vi "UI Controller.vi"(8 "Error In":errorcluster) -> (0 "Error Out":errorcluster)   [LabVIEW 2019, in "Controller.lvlib"]
uses:
  Controller.lvlib
  User Event/Controls/UE Abort Action.ctl
  <vilib>/Utility/miscctls.llb/LVPointTypeDef.ctl
  Queues/Queues.lvlib
  Initialize/Initialize.lvlib
  UI/UI Main Page.vi
  UI/UIs.lvlib
panel:
  out "String":string
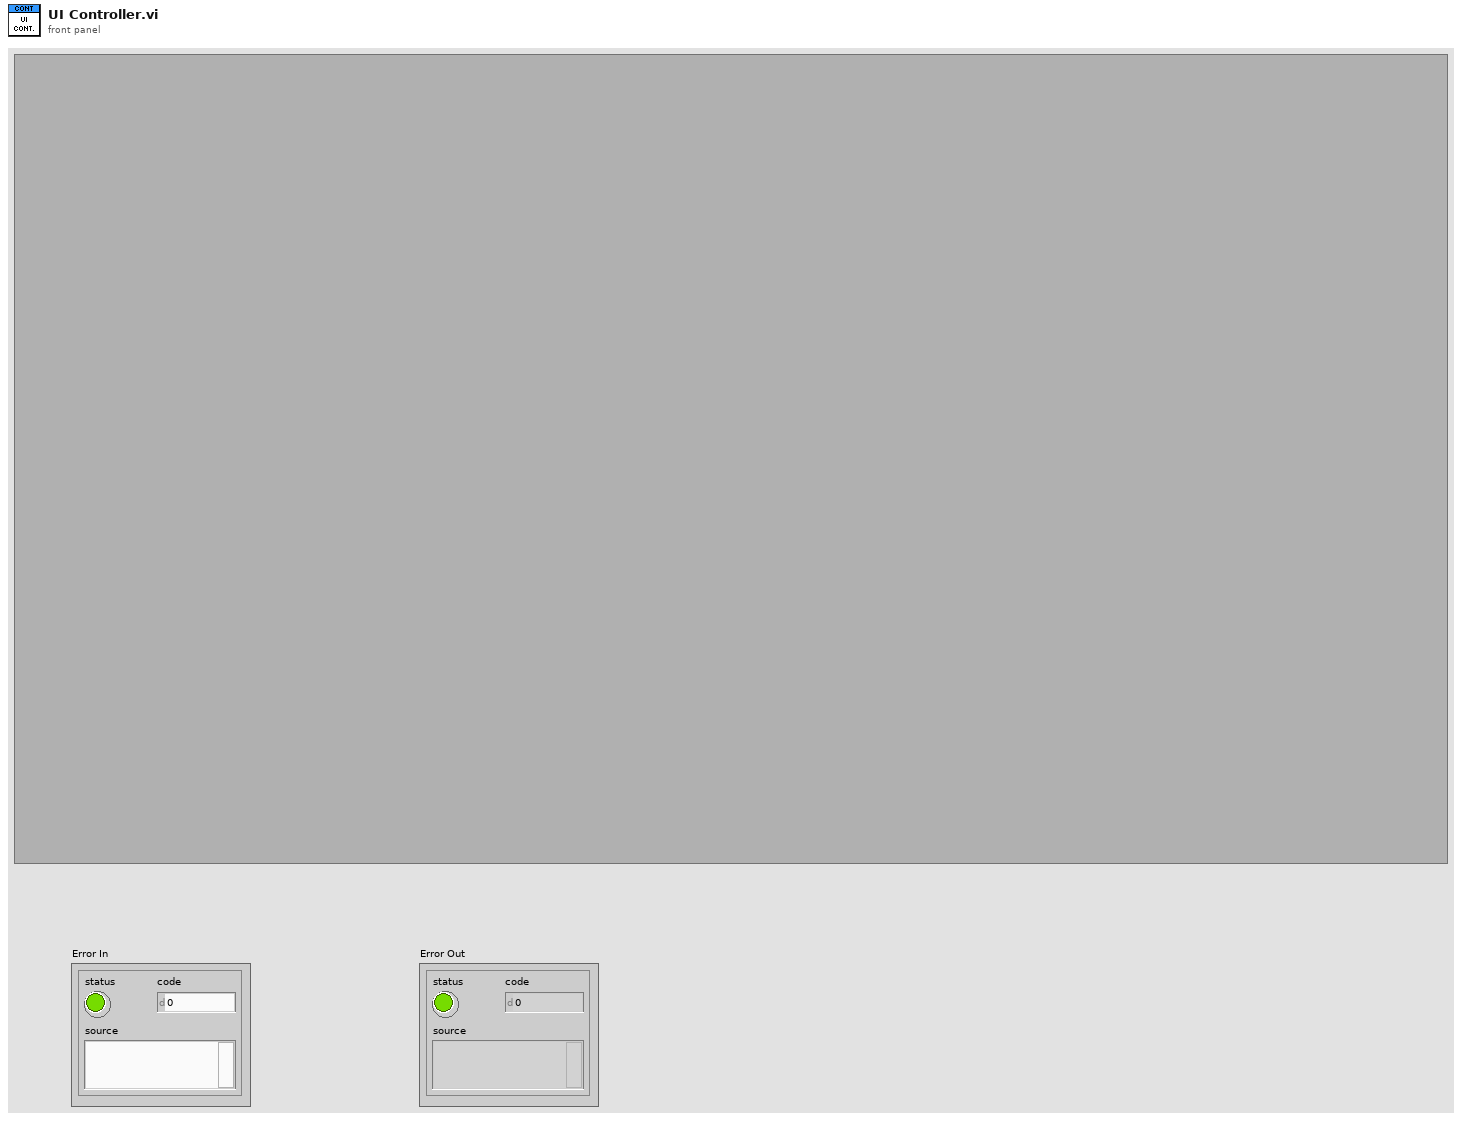
[diagram p1: front panel]
types:
  T1 = typedef "UE Abort Action.ctl" = enum16{"Create", "Get", "Destroy"}
  T2 = typedef "LVPointTypeDef.ctl" = cluster{"Horizontal":i16, "Vertical":i16}
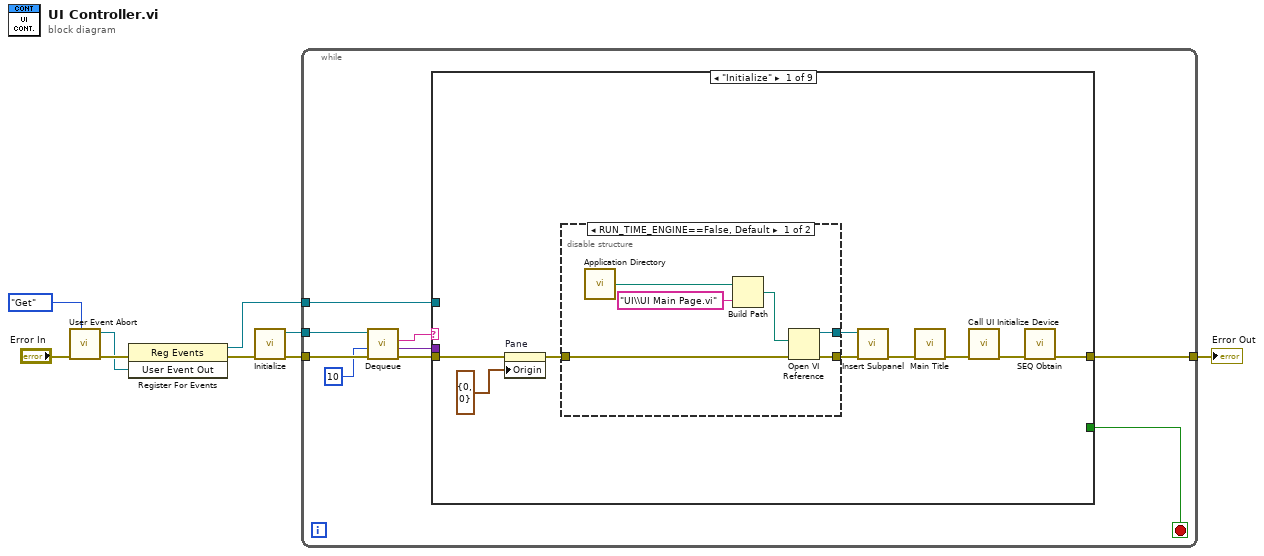
[diagram p0: block diagram]
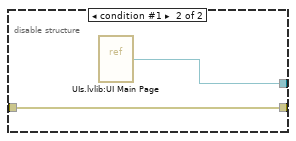
[diagram p2: hidden frame]
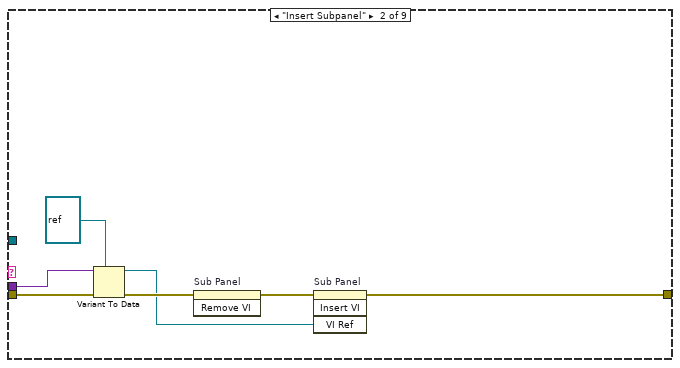
[diagram p3: hidden frame]
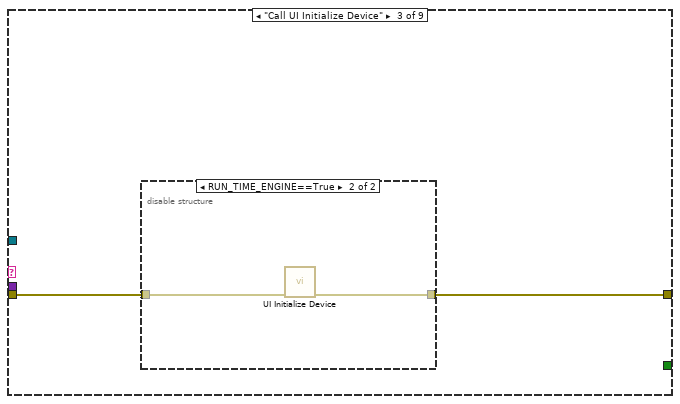
[diagram p4: hidden frame]
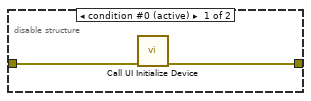
[diagram p5: hidden frame]
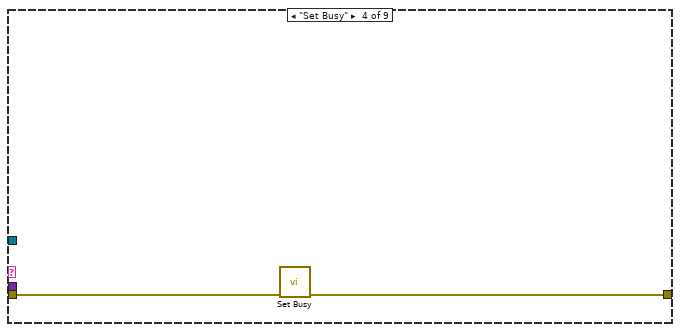
[diagram p6: hidden frame]
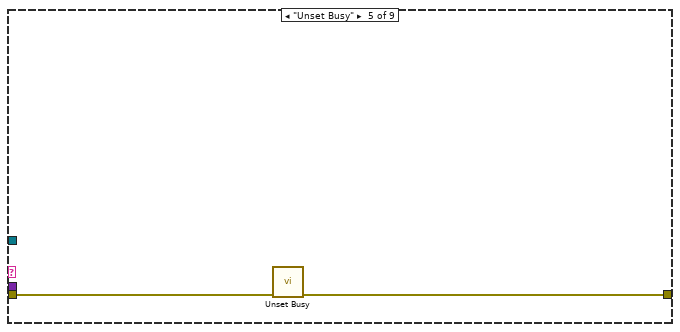
[diagram p7: hidden frame]
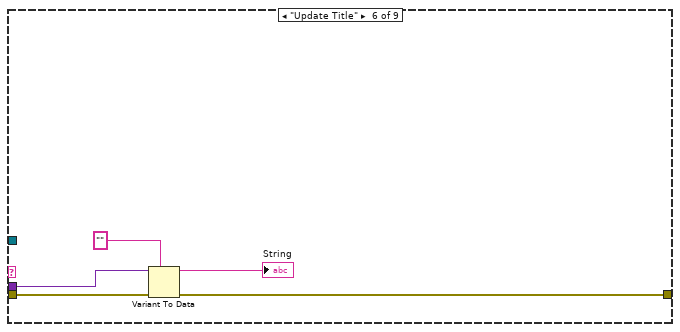
[diagram p8: hidden frame]
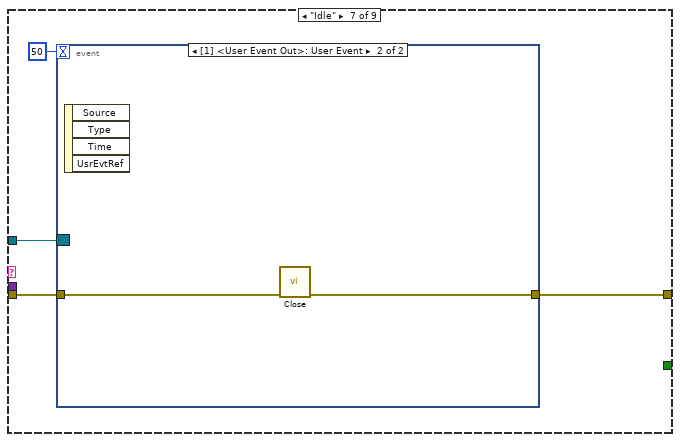
[diagram p9: hidden frame]
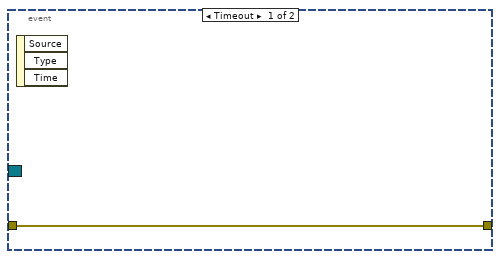
[diagram p10: hidden frame]
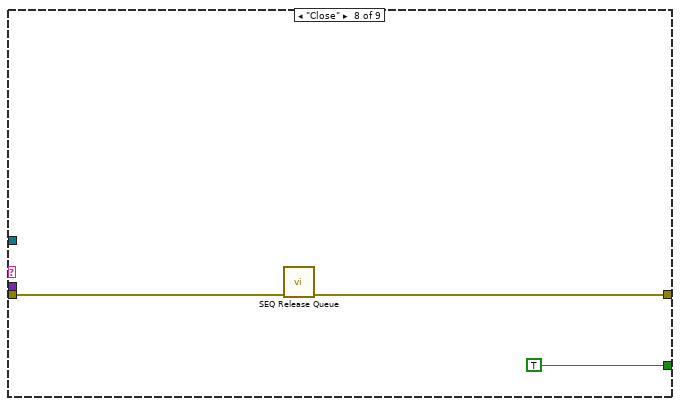
[diagram p11: hidden frame]
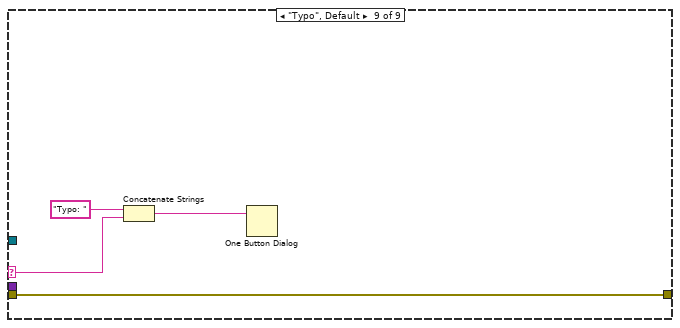
[diagram p12: hidden frame]
diagram:
  n1 = call "User Event Abort.vi"("Action"=UE_Abort_Action."Get", "Error In"="Error In") -> ("Error Out"=w4:errorcluster, "User Event Out"=w3:refnum<user-event>)  [unwired: 8 in]
  n2 = register-events(error in=w4, w3) -> (reference out=w1:refnum<event-registration>, error out=w2:errorcluster)  [unwired: 1 in]
  n3 = call "Initialize.vi"("Error In"=w2) -> ("Error Out"=w8:errorcluster, "Queue out"=w7:refnum<queue>)  [unwired: 9 in]
  n4 = while {
    tunnel: w7 -> [w18]
    tunnel: w8 -> [w17]
    tunnel: [w12] -> w9
    tunnel: w1 -> [w11]
    stop <- w10 stop-if-true
    n5 = call "Dequeue.vi"("Error In"=w17, "timeout in ms (-1)"=10, "Queue in"=w18) -> ("Error Out"=w16:errorcluster, "Data"=w14:variant, "State"=w15:string)  [unwired: 5 in, 1 out]
    n6 = case shown="\"Initialize\"" w15 {
      selector: w15 -> [_ _ _ _ _ _ _ _ w70]
      tunnel: w16 -> [w26 w42 w44 w50 w52 w57 w61 w66 w71]
      tunnel: [w21 w39 w43 w49 w51 w55 w59 w65 w71] -> w12
      tunnel: w14 -> [_ w38 _ _ _ w56 _ _ _]
      tunnel: w11 -> [_ _ _ _ _ _ w58 _ _]
      tunnel: [_ _ _ _ _ _ _ TRUE _] -> w10
      frame "Initialize" {
        n7 = property on="Pane" class="Pane"(error in=w26, "Origin"=T2 {"Horizontal"=0, "Vertical"=0}) -> (error out=w23:errorcluster)  [unwired: 1 in, 1 out]
        n8 = disable-structure shown="RUN_TIME_ENGINE==False, Default" {
          disable-tunnel: [w32 w34] -> w25
          disable-tunnel: [w31 w35] -> w24
          disable-tunnel: w23 -> [w30 w34]
          frame condition #0 (active) {
            n9 = call <vilib>:"Application Directory.vi"() -> ("Application Directory"=w29:path)
            n10 = Build Path(base path=w29, name or relative path="UI\\UI Main Page.vi") -> (appended path=w33:path)
            n11 = Open VI Reference(vi path=w33, error in (no error)=w30) -> (vi reference=w31:refnum<vi>, error out=w32:errorcluster)  [unwired: 4 in]
          }
          frame condition #1 {
            n12 = vi-ref "UIs.lvlib:UI Main Page.vi"() -> (w35:refnum<vi>)
          }
        }
        n13 = call "Insert Subpanel.vi"("Error In"=w25, "VI Refnum"=w24) -> ("Error Out"=w20:errorcluster)  [unwired: 9 in]
        n14 = call "Main Title.vi"("Error In"=w20) -> ("Error Out"=w19:errorcluster)  [unwired: 10 in]
        n15 = call "Call UI Initialize Device.vi"("Error In"=w19) -> ("Error Out"=w22:errorcluster)  [unwired: 10 in]
        n16 = call "SEQ Obtain.vi"("error in"=w22) -> ("error out"=w21:errorcluster)  [unwired: 9 in, 1 out]
      }
      frame "Insert Subpanel" {
        n17 = Variant To Data(error in=w42, type=refnum<vi> refnum ("VI Ref"), Variant=w38) -> (data=w36:refnum<vi>, error out=w41:errorcluster)
        n18 = invoke on="Sub Panel" class="SubPnl" method="Remove VI"(error in=w41) -> (error out=w40:errorcluster)  [unwired: 2 in, 2 out]
        n19 = invoke on="Sub Panel" class="SubPnl" method="Insert VI"(error in=w40, "VI Ref"=w36) -> (error out=w39:errorcluster)  [unwired: 2 in, 3 out]
      }
      frame "Call UI Initialize Device" {
        n20 = disable-structure shown="RUN_TIME_ENGINE==True" {
          disable-tunnel: w44 -> [w46 w48]
          disable-tunnel: [w45 w47] -> w43
          frame condition #0 (active) {
            n21 = call "Call UI Initialize Device.vi"("error in"=w46) -> ("error out"=w45:errorcluster)  [unwired: 10 in]
          }
          frame condition #1 {
            n22 = call "UI Initialize Device.vi"("error in"=w48) -> ("error out"=w47:errorcluster)  [unwired: 10 in]
          }
        }
      }
      frame "Set Busy" {
        n23 = call <vilib>:"Set Busy.vi"("error in (no error)"=w50) -> ("error out"=w49:errorcluster)  [unwired: 9 in, 1 out]
      }
      frame "Unset Busy" {
        n24 = call <vilib>:"Unset Busy.vi"("error in (no error)"=w52) -> ("error out"=w51:errorcluster)  [unwired: 10 in]
      }
      frame "Update Title" {
        n25 = Variant To Data(error in=w57, type="", Variant=w56) -> (data=→"String":string, error out=w55:errorcluster)
      }
      frame "Idle" {
        n26 = event shown="[1] <User Event Out>: User Event" {
          selector: w58 -> [_ _]
          dyn-events: _ -> [_ _]
          timeout: 50 -> [_ _]
          tunnel: w61 -> [w62 w64]
          tunnel: [w62 w63] -> w59
          event Timeout {
            n27 = event-data() -> ()  [unwired: 1 in, 3 out]
          }
          event User Event {
            n28 = event-data() -> ()  [unwired: 1 in, 4 out]
            n29 = call "Close.vi"("Error In"=w64) -> ("Error Out"=w63:errorcluster)  [unwired: 10 in]
          }
        }
      }
      frame "Close" {
        n30 = call "SEQ Release Queue.vi"("error in"=w66) -> ("error out"=w65:errorcluster)  [unwired: 10 in]
      }
      frame "Typo", Default {
        n31 = Concatenate Strings("Typo: " ("string"), w70) -> (w68:string)
        n32 = One Button Dialog(message=w68) -> ()  [unwired: 1 in, 1 out]
      }
    }
  }
  "Error Out" <- w9
